vi "Start cRIO fast measure.vi"(8 "error in (no error)":errorcluster, 11 "machine IP":string="172.22.11.2") -> (0 "error out":errorcluster, 2 "vi reference":refnum<vi>, 3 "application reference":refnum<vi>)   [LabVIEW 2023]
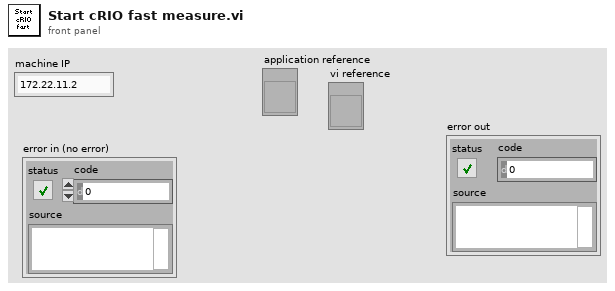
[diagram p1: front panel]
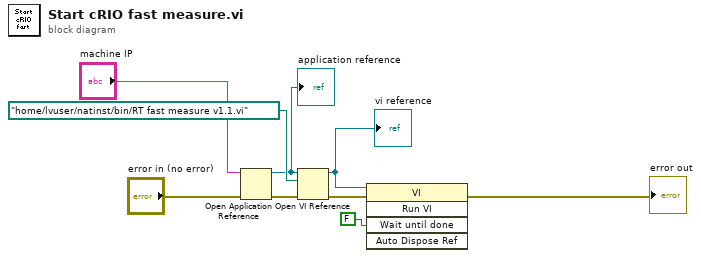
[diagram p0: block diagram]
diagram:
  n1 = Open Application Reference(8:"error in (no error)", 11:"machine IP") -> (0:w7:errorcluster, 3:w1:refnum<vi>)  [unwired: 2 in]
  "application reference" <- w1
  n2 = Open VI Reference(application reference (local)=w1, vi path=path "/home/lvuser/natinst/bin/RT fast measure v1.1.vi", error in (no error)=w7) -> (vi reference=w4:refnum<vi>, error out=w3:errorcluster)  [unwired: 3 in]
  "vi reference" <- w4
  n3 = invoke class="VI" method="Run VI"(reference=w4, error in=w3, "Wait until done"=FALSE ("Wait Until Done")) -> (error out=→"error out":errorcluster)  [unwired: 2 in, 4 out]
